vi "7a_Numeric_Case(170382,170307).vi"() -> ()   [LabVIEW 2015]
panel:
  in  "Numeric":u32
  in  "Menu Ring":u16(ring) items=["Add", "Subtract", "Multiply", "Divide"]
  in  "stop":bool
  in  "Listbox":i32(listbox)
  out "Result":dbl
  in  "B":dbl
  in  "A":dbl
  # "Do not run this in continuous mode"
  # "Connect one of these at a time to the selector terminal."
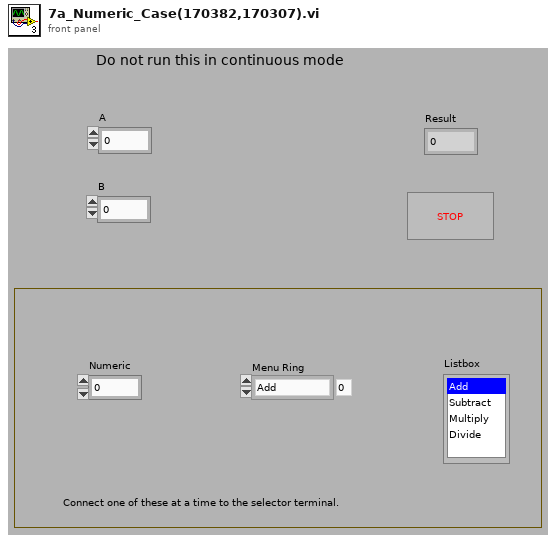
[diagram p1: front panel]
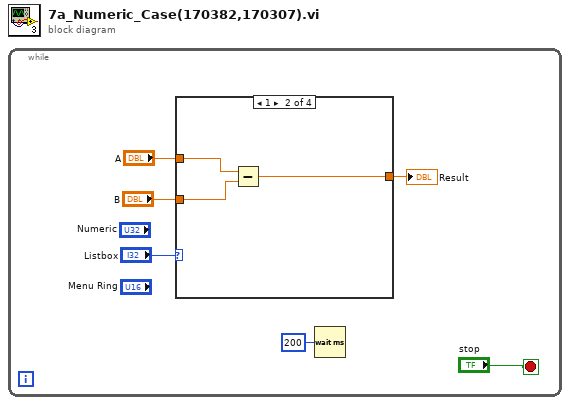
[diagram p0: block diagram]
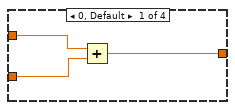
[diagram p2: hidden frame]
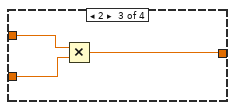
[diagram p3: hidden frame]
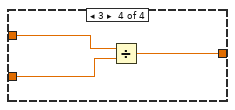
[diagram p4: hidden frame]
diagram:
  n1 = while {
    stop <- "stop" stop-if-true
    n2 = case shown="1" "Listbox" {
      tunnel: "B" -> [w8 w11 w13 w16]
      tunnel: "A" -> [w9 w10 w14 w17]
      tunnel: [w7 w12 w15 w18] -> w4
      frame 0, Default {
        n3 = Add(x=w9, y=w8) -> (x+y=w7:dbl)
      }
      frame 1 {
        n4 = Subtract(x=w10, y=w11) -> (x-y=w12:dbl)
      }
      frame 2 {
        n5 = Multiply(x=w14, y=w13) -> (x*y=w15:dbl)
      }
      frame 3 {
        n6 = Divide(x=w17, y=w16) -> (x/y=w18:dbl)
      }
    }
    "Result" <- w4
    n7 = Wait (ms)(milliseconds to wait=u32 200) -> ()  [unwired: 1 out]
  }
